vi "Outputs SW Set.vi"(7 "Current Time":timestamp format="%<%x %.3X>T", 8 "HW Config":T1={"SholderHW Ver"=0, "CAN"={"ID"=0, "Bus"=""}, "Output"={"Type"=enum."Counter-Clockwise", "Neutral"=enum."Override to Coast", "Max"={"FWD"=1.0, "REV"=-1.0}, "Min"={"FWD"=0.0, "REV"=0.0}, "OL Ramp Rate (S)"=0.0, "Dead Band"=0.0}, "CL"={"Gains"={"P"=1.0, "I"=0.01, "D"=0.0, "F"=0.0}, "Error Allowed"={"High"=0.0, "Low"=0.0}, "I Zone"={"High"=10000.0, "Low"=-1000.0}, "Max Out"={"FWD"=1.0, "REV"=-1.0}, "Max I Accu"={"High"=10.0, "Low"=-10.0}, "CL Ramp Rate (S)"=0.0}, "MM"={"Cruise Velocity"=5000, "Acceleration"=5000}, "TravelLimits"={"Hard"={"FWD Switch Normal"=enum."Normally Open", "FWD On will Zero Encoder "=FALSE, "REV Switch Normal"=enum."Normally Open", "REV On will Zero Encoder "=FALSE}, "Soft"={"FWD"={"Enable"=FALSE, "Counts"=0}, "REV"={"Enable"=FALSE, "Counts"=0}}}, "Cancoder"={"ID"=0, "CW(t) CCW(f)"=TRUE, "Zero Offset"=0.0}} {"TravelLimits"."Soft"."REV"."Counts" format="%#.0f"; "TravelLimits"."Soft"."FWD"."Counts" format="%#.0f"; "Output"."Min"."REV" format="%.2f"; "Output"."Min"."FWD" format="%.2f"; "Output"."Max"."REV" format="%.2f"; "Output"."Max"."FWD" format="%.2f"; "CL"."Max I Accu"."Low" format="%#.8f"; "CL"."Max I Accu"."High" format="%#.8f"; "CL"."Gains"."F" format="%#.8f"; "CL"."Gains"."D" format="%#.8f"; "CL"."Gains"."I" format="%#.8f"; "CL"."Gains"."P" format="%#.8f"; "CL"."Error Allowed"."Low" format="%#.8f"; "CL"."Error Allowed"."High" format="%#.8f"; "CL"."I Zone"."Low" format="%#.8f"; "CL"."I Zone"."High" format="%#.8f"; "CL"."Max Out"."REV" format="%.2f"; "CL"."Max Out"."FWD" format="%.2f"}, 9 "SW Config":T17={"SholderSW Ver"=0, "At Position Delay(S)"=0.2}, 10 "Outputs FX":T19, 11 "SW Output":T18) -> (3 "SW Output Out":T18)   [LabVIEW 2020, in "Sholder_ACT.lvlib"]
uses:
  Sholder_ACT.lvlib
  Shared Code/TypeDefs/Cluster_Sholder_HW Outputs.ctl
  Shared Code/TypeDefs/Cluster_FX Sensor Values.ctl
  Shared Code/TypeDefs/Cluster_FX CloseLoop Values.ctl
  Shared Code/TypeDefs/Cluster_FX Limit Switchs.ctl
  Shared Code/TypeDefs/Cluster_FX Current Values.ctl
  Shared Code/TypeDefs/Cluster_FX Integrated Sensor Values.ctl
  Shared Code/TypeDefs/Cluster_Sholder_SW Output Data.ctl
  Shared Code/TypeDefs/Cluster_Sholder_Config SW Values.ctl
  Shared Code/TypeDefs/Cluster_Sholder_Config HW Values.ctl
  Shared Code/TypeDefs/Cluser_CAN Data.ctl
  Shared Code/TypeDefs/Cluster_Config Motor Output.ctl
  <vilib>/Rock Robotics/WPI/ThirdParty/Phoenix-LabVIEW/Motor Controller/Controls/CTRE_Phoenix_MotorControl_TalonFXInvertType.ctl
  <vilib>/Rock Robotics/WPI/ThirdParty/Phoenix-LabVIEW/Motor Controller/Controls/CTRE_Phoenix_MotorControl_NeutralMode.ctl
  Shared Code/TypeDefs/Cluster_FWD  REV Values.ctl
  Shared Code/TypeDefs/Cluster_PID Config.ctl
  Shared Code/TypeDefs/Cluster_PID Gains.ctl
  Shared Code/TypeDefs/Cluster_High-Low.ctl
  Shared Code/TypeDefs/Cluster_Motion Magic Parameters.ctl
  Shared Code/TypeDefs/Cluser_Limit Travel Config.ctl
  Shared Code/TypeDefs/Cluser_Hard Limits.ctl
  <vilib>/Rock Robotics/WPI/ThirdParty/Phoenix-LabVIEW/Motor Controller/Controls/CTRE_Phoenix_MotorControl_LimitSwitchNormal.ctl
  Shared Code/TypeDefs/Cluser_Config_Soft Limits.ctl
  Shared Code/TypeDefs/Cluser_Enable-Value I32.ctl
  Shared Code/TypeDefs/Cluster_Config_Cancoder Data.ctl
panel:
  # "Tune Output\nto 1023 Max"
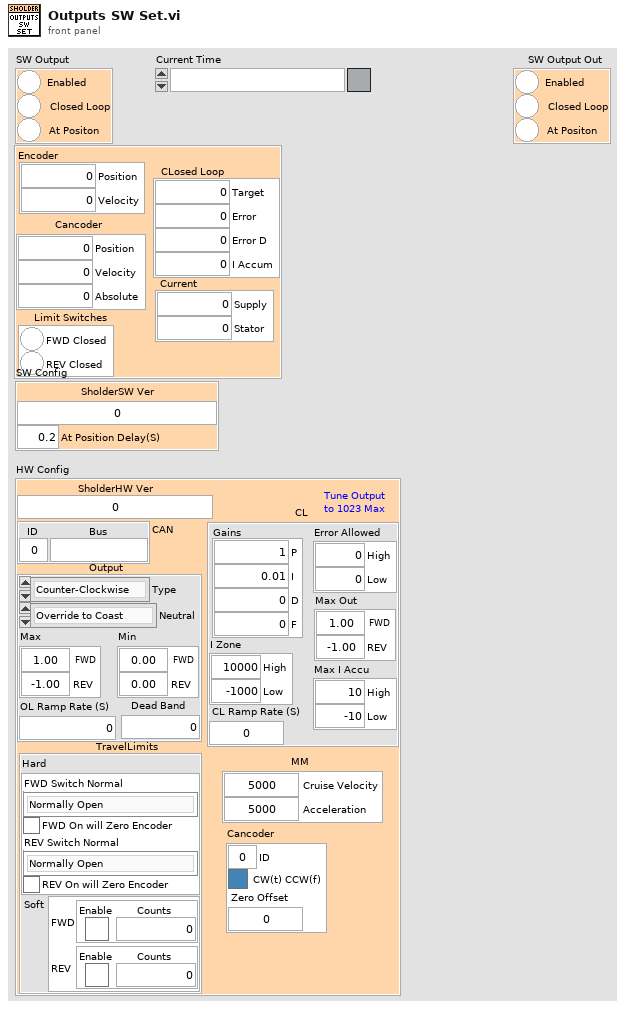
[diagram p1: front panel]
types:
  T1 = typedef "Cluster_Sholder_Config HW Values.ctl" = cluster{"SholderHW Ver":u64, "CAN":T2, "Output":T3, "CL":T7, "MM":T10, "TravelLimits":T11, "Cancoder":T16}
  T2 = typedef "Cluser_CAN Data.ctl" = cluster{"ID":u8, "Bus":string}
  T3 = typedef "Cluster_Config Motor Output.ctl" = cluster{"Type":T4, "Neutral":T5, "Max":T6, "Min":T6, "OL Ramp Rate (S)":dbl, "Dead Band":dbl}
  T4 = typedef "CTRE_Phoenix_MotorControl_TalonFXInvertType.ctl" = enum16{"Counter-Clockwise", "Clockwise"}
  T5 = typedef "CTRE_Phoenix_MotorControl_NeutralMode.ctl" = enum8{"EEPROMSetting", "Override to Coast", "Override to Brake"}
  T6 = typedef "Cluster_FWD  REV Values.ctl" = cluster{"FWD":dbl, "REV":dbl}
  T7 = typedef "Cluster_PID Config.ctl" = cluster{"Gains":T8, "Error Allowed":T9, "I Zone":T9, "Max Out":T6, "Max I Accu":T9, "CL Ramp Rate (S)":dbl}
  T8 = typedef "Cluster_PID Gains.ctl" = cluster{"P":dbl, "I":dbl, "D":dbl, "F":dbl}
  T9 = typedef "Cluster_High-Low.ctl" = cluster{"High":dbl, "Low":dbl}
  T10 = typedef "Cluster_Motion Magic Parameters.ctl" = cluster{"Cruise Velocity":i32, "Acceleration":i32}
  T11 = typedef "Cluser_Limit Travel Config.ctl" = cluster{"Hard":T12, "Soft":T14}
  T12 = typedef "Cluser_Hard Limits.ctl" = cluster{"FWD Switch Normal":T13, "FWD On will Zero Encoder ":bool, "REV Switch Normal":T13, "REV On will Zero Encoder ":bool}
  T13 = typedef "CTRE_Phoenix_MotorControl_LimitSwitchNormal.ctl" = enum16{"Normally Open", "Normally Closed", "Disabled"}
  T14 = typedef "Cluser_Config_Soft Limits.ctl" = cluster{"FWD":T15, "REV":T15}
  T15 = typedef "Cluser_Enable-Value I32.ctl" = cluster{"Enable":bool, "Counts":i32}
  T16 = typedef "Cluster_Config_Cancoder Data.ctl" = cluster{"ID":u8, "CW(t) CCW(f)":bool, "Zero Offset":dbl}
  T17 = typedef "Cluster_Sholder_Config SW Values.ctl" = cluster{"SholderSW Ver":u64, "At Position Delay(S)":dbl}
  T18 = typedef "Cluster_Sholder_SW Output Data.ctl" = cluster{"Enabled":bool, "Closed Loop":bool, "At Positon":bool}
  T19 = typedef "Cluster_Sholder_HW Outputs.ctl" = cluster{"Encoder":T20, "CLosed Loop":T21, "Limit Switches":T22, "Current":T23, "Cancoder":T24}
  T20 = typedef "Cluster_FX Sensor Values.ctl" = cluster{"Position":i32, "Velocity":i32}
  T21 = typedef "Cluster_FX CloseLoop Values.ctl" = cluster{"Target":dbl, "Error":i32, "Error D":dbl, "I Accum":dbl}
  T22 = typedef "Cluster_FX Limit Switchs.ctl" = cluster{"FWD Closed":bool, "REV Closed":bool}
  T23 = typedef "Cluster_FX Current Values.ctl" = cluster{"Supply":dbl, "Stator":dbl}
  T24 = typedef "Cluster_FX Integrated Sensor Values.ctl" = cluster{"Position":dbl, "Velocity":dbl, "Absolute":dbl}
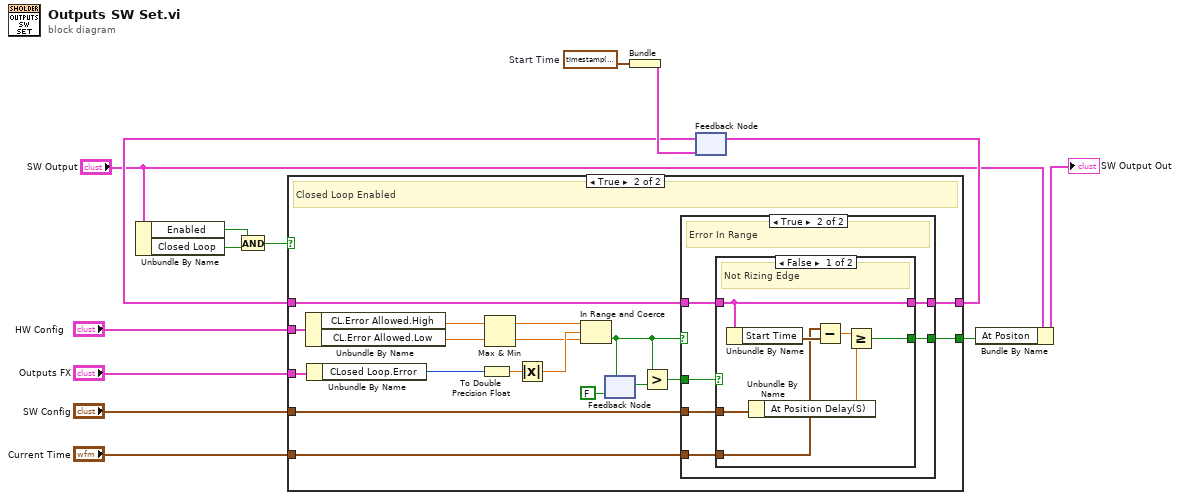
[diagram p0: block diagram]
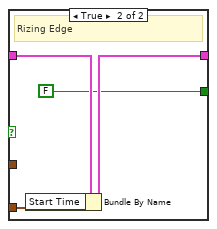
[diagram p4: hidden frame]
diagram:
  w8 = timestamp(0 s since 1904-01-01)  # Start Time
  n1 = Unbundle By Name("SW Output") -> ("Enabled"=w14:bool, "Closed Loop"=w13:bool)
  n2 = And(x=w14, y=w13) -> (x .and. y?=w9:bool)
  n3 = Bundle("Start Time"=w8) -> (w7:cluster{"Start Time":timestamp})  [unwired: 1 in]
  n4 = feedback #1(w7) -> (w6:cluster{"Start Time":timestamp})
  n5 = case shown="True" w9 {
    tunnel: "SW Config" -> [_ w33]
    tunnel: "Outputs FX" -> [_ w31]
    tunnel: "Current Time" -> [_ w21]
    tunnel: w6 -> [w15 w32]
    tunnel: [w15 w22] -> w5
    tunnel: [_ w20] -> w2
    tunnel: "HW Config" -> [_ w30]
    frame False {
    }
    frame True {
      # "Closed Loop Enabled"
      n6 = Unbundle By Name(w30) -> ("CL.Error Allowed.High"=w29:dbl, "CL.Error Allowed.Low"=w18:dbl)
      n7 = Unbundle By Name(w31) -> ("CLosed Loop.Error"=w28:i32)
      n8 = To Double Precision Float(number=w28) -> (double precision float=w27:dbl)
      n9 = Max & Min(x=w29, y=w18) -> (max(x,y)=w19:dbl, min(x,y)=w16:dbl)
      n10 = Absolute Value(x=w27) -> (abs(x)=w17:dbl)
      n11 = In Range and Coerce(upper limit=w19, x=w17, lower limit=w16) -> (In Range?=w24:bool)  [unwired: 1 out]
      n12 = feedback #2(FALSE) -> (w26:bool)
      n13 = feedback-in #2(w24) -> ()
      n14 = Greater?(x=w24, y=w26) -> (0:w23:bool)
      n15 = case shown="True" w24 {
        selector: w24 -> [w34 _]
        tunnel: w33 -> [_ w41]
        tunnel: w32 -> [w35 w39]
        tunnel: w23 -> [_ w40]
        tunnel: [w35 w38] -> w22
        tunnel: w21 -> [_ w37]
        tunnel: [w34 w36] -> w20
        frame False {
          # "Error Out of Range"
        }
        frame True {
          # "Error In Range"
          n16 = case shown="False" w40 {
            tunnel: w41 -> [w44 _]
            tunnel: w39 -> [w48 w50]
            tunnel: [w48 w51] -> w38
            tunnel: w37 -> [w46 w52]
            tunnel: [w42 FALSE] -> w36
            frame False {
              # "Not Rizing Edge"
              n17 = Unbundle By Name(w48) -> ("Start Time"=w47:timestamp)
              n18 = Unbundle By Name(w44) -> ("At Position Delay(S)"=w43:dbl)
              n19 = Subtract(x=w46, y=w47) -> (x-y=w45:dbl)
              n20 = Greater Or Equal?(x=w45, y=w43) -> (x >= y?=w42:bool)
            }
            frame True {
              # "Rizing Edge"
              n21 = Bundle By Name(cluster=w50, "Start Time"=w52) -> (w51:cluster{"Start Time":timestamp})
            }
          }
        }
      }
    }
  }
  n22 = feedback-in #1(w5) -> ()
  n23 = Bundle By Name(cluster="SW Output", "At Positon"=w2) -> (→"SW Output Out":T18)
